vi "SPM Pump v0.1.vi"(0 "Delay before read (ms)":u32=1000, 1 "string to write":string="/1ZR", 2 "Time <input>":string, 3 "byte count":u32=64, 4 "Timeout (ms)":u32=10000, 5 "error in (no error)":errorcluster, 6 "Termination char\n(0xA = '\\n' = LF)\n(0xD = '\\r' = CR)":u8=13 format="%.0x", 7 "VISA resource name":refnum<visa-resource-name>="COM6", 10 "Enable Termination\nChar (T)":bool=TRUE, 11 "baud rate":u32=9600, 12 "parity":u16(ring) items=["None", "Odd", "Even", "Mark", "Space"], 13 "data bits":u16=8 min=5 max=8 step=1, 14 "stop bits":u16(ring)=10 items=["1.0"=10, "1.5"=15, "2.0"=20], 15 "flow control":u16(ring) items=["None"=0, "XON/XOFF"=1, "RTS/CTS"=2, "DTR/DSR"=4], 16 "Serial Settings:Serial End Mode for Reads":u16(ring)=2 items=["None", "LastBit", "TermChar"]) -> (8 "Error bit":string, 9 "Response":string, 18 "Serial port output":string, 19 "error out":errorcluster)   [LabVIEW 2016]
doc: "The Basic Serial Read and Write example performs a Serial Port Read, a Serial Port Write, or a combination of these actions. The user selects the actions (read or write) on the front panel. If both are selected, the VI will write the data first, read data, and then close the VISA session that is opened to the port. This VI will wait until the specified number of bytes is received at the port. Only the number of bytes specified will be read.\n\nINSTRUCTIONS:\n1) Select the serial resource and configuration parameters (baud rate, data bits, parity, stop bits, flow control).\n2) Select the operations to be performed. \n3) Connect the serial port to your device. If no device is available, perform a loopback test by doing one of the following. Short pins 2 and 3 on a RS-232 cable or short pin 4 to pin 8 and pin 5 to pin 9 on a RS-485/422 cable. \n4) Run the VI to see the data read. (The \"read string\" will match the \"string to write\" if a loopback test was performed.)\n\nNote: The parameters set for the serial port must match the parameters of the connected instrument or device. In this example, the bytes to read parameter specifies the number of bytes that the serial port reads. If there were more bytes at the port than the number specified in bytes to read, those bytes would not be read. Also, if you specify to read more bytes than the number of bytes actually read, you might receive a timeout error message.\n\nOn the block diagram, the Configure Serial Port VI sets the configuration parameters. The front panel displays the controls used to configure the basic parameters, such as baud rate, data bits, and parity. Constants configure the other parameters the user probably does not need set. After the VISA Configure Serial Port VI opens the VISA session and configures the port, the VI passes the VISA resource name to other VIs that perform operations on that VISA resource. The VISA Write function sends a command to the serial device and the VISA Read function returns data based on the command. The VISA Close function then closes the reference to the serial device. It is important to close the reference; otherwise communication through with that port through protocols other than VISA might not be possible."
panel:
  # "Select the serial resource and the operations (Read, Write, or both) to be performed.  If both are selected, the VI will write the data first, read data and then close the VISA session that is opened to the port.  This VI will wait until the specified number of bytes is received at the port. Only the number of bytes specified will be read."
  # "For additional information select File >> VI Properties >> Documentation"
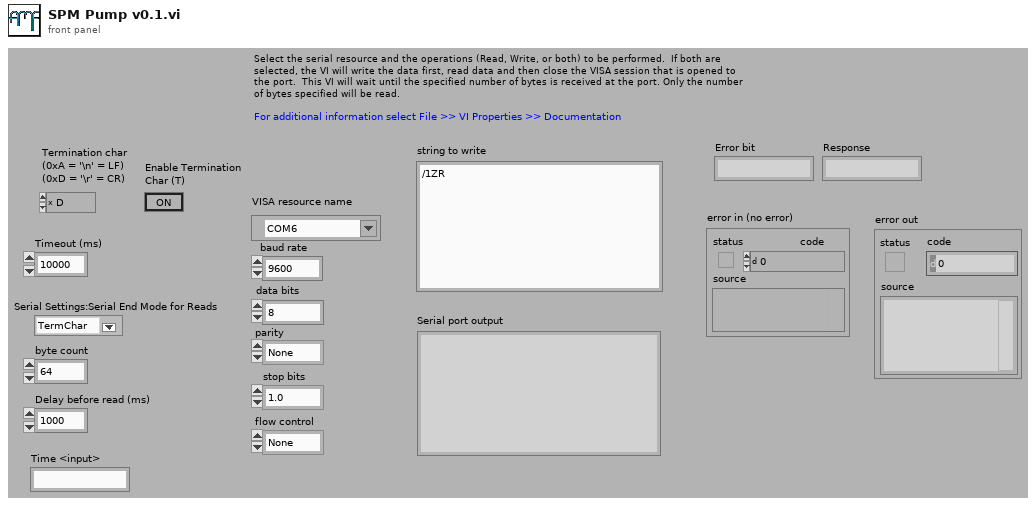
[diagram p1: front panel]
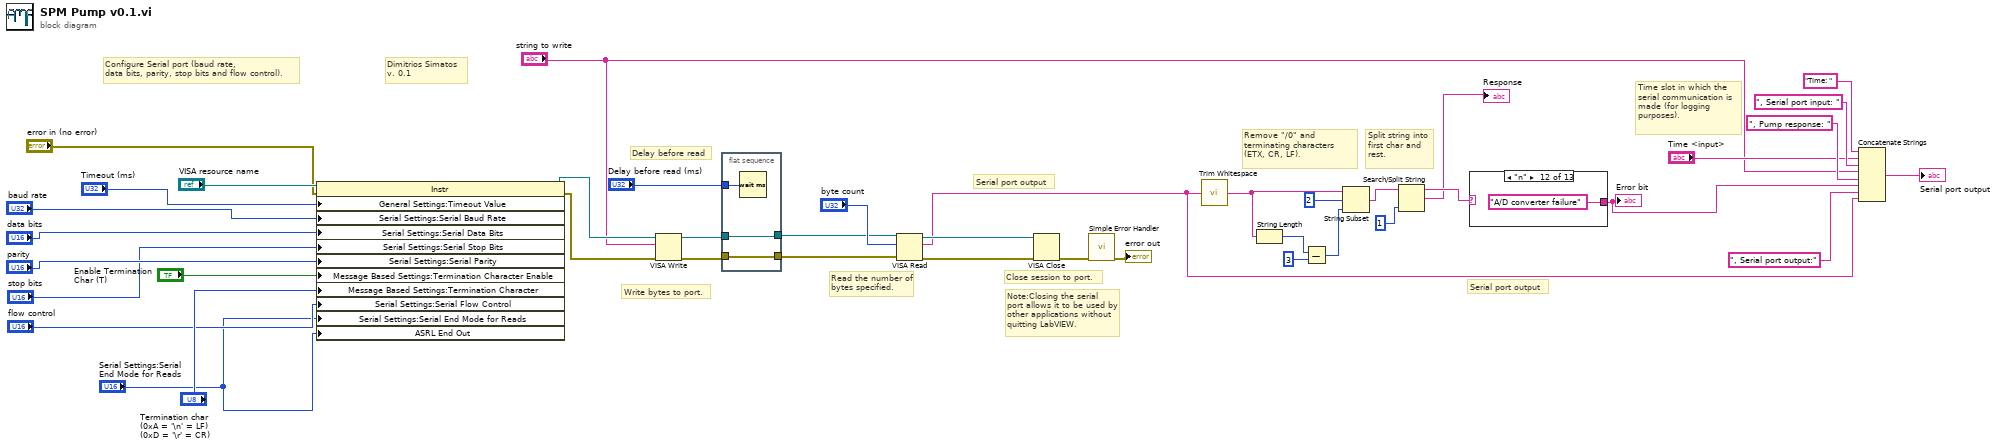
[diagram p0: block diagram]
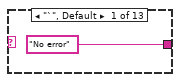
[diagram p2: hidden frame]
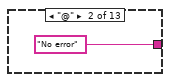
[diagram p3: hidden frame]
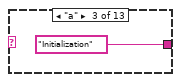
[diagram p4: hidden frame]
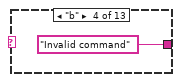
[diagram p5: hidden frame]
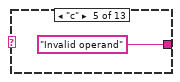
[diagram p6: hidden frame]
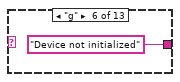
[diagram p7: hidden frame]
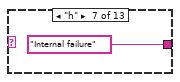
[diagram p8: hidden frame]
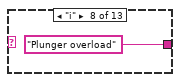
[diagram p9: hidden frame]
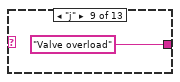
[diagram p10: hidden frame]
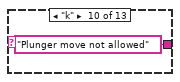
[diagram p11: hidden frame]
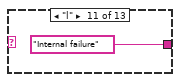
[diagram p12: hidden frame]
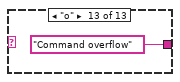
[diagram p13: hidden frame]
diagram:
  # "Serial port output"
  # "Serial port output"
  # "Time slot in which the serial communication is made (for logging purposes)."
  # "Split string into first char and rest."
  # "Remove \"/0\" and terminating characters (ETX, CR, LF)."
  # "Delay before read"
  # "Dimitrios Simatos\nv. 0.1"
  # "Read the number of bytes specified."
  # "Write bytes to port."
  # "Note:Closing the serial port allows it to be used by other applications without\nquitting LabVIEW."
  # "Configure Serial port (baud rate,\ndata bits, parity, stop bits and flow control)."
  # "Close session to port."
  n1 = property class="Instr"(reference="VISA resource name", error in="error in (no error)", "General Settings:Timeout Value"="Timeout (ms)", "Serial Settings:Serial Baud Rate"="baud rate", "Serial Settings:Serial Data Bits"="data bits", "Serial Settings:Serial Stop Bits"="stop bits", "Serial Settings:Serial Parity"="parity", "Message Based Settings:Termination Character Enable"="Enable Termination\nChar (T)", "Message Based Settings:Termination Character"="Termination char\n(0xA = '\\n' = LF)\n(0xD = '\\r' = CR)", "Serial Settings:Serial Flow Control"="flow control", "Serial Settings:Serial End Mode for Reads"="Serial Settings:Serial End Mode for Reads", "ASRL End Out"="Serial Settings:Serial End Mode for Reads") -> (reference out=w28:refnum<visa-resource-name>, error out=w27:errorcluster)
  n2 = VISA Write(VISA resource name=w28, write buffer="string to write", error in (no error)=w27) -> (VISA resource name out=w23:refnum<visa-resource-name>, error out=w22:errorcluster)  [unwired: 1 out]
  n3 = flat-sequence {
    tunnel: w22 -> [w43]
    tunnel: [w43] -> w21
    tunnel: w23 -> [w42]
    tunnel: [w42] -> w20
    tunnel: "Delay before read (ms)" -> [w44]
    frame #0 {
      n4 = Wait (ms)(milliseconds to wait=w44) -> ()  [unwired: 1 out]
    }
  }
  n5 = VISA Read(VISA resource name=w20, byte count="byte count", error in (no error)=w21) -> (VISA resource name out=w40:refnum<visa-resource-name>, read buffer=w3:string, error out=w41:errorcluster)  [unwired: 1 out]
  n6 = VISA Close(VISA resource name=w40, error in (no error)=w41) -> (error out=w39:errorcluster)
  n7 = call <vilib>:"Simple Error Handler.vi"("error in (no error)"=w39) -> ("error out"=→"error out":errorcluster)  [unwired: 4 in, 4 out]
  n8 = call <vilib>:"Trim Whitespace.vi"("string"=w3) -> ("trimmed string"=w14:string)  [unwired: 1 in]
  n9 = String Length(string=w14) -> (length=w18:i32)
  n10 = Subtract(x=w18, y=3) -> (x-y=w17:i32)
  n11 = String Subset(string=w14, offset (0)=2, length (rest)=w17) -> (substring=w13:string)
  n12 = Search/Split String(string=w13, offset (0)=1) -> (substring before match=w11:string, match + rest of string=→"Response":string)  [unwired: 1 in, 1 out]
  n13 = case shown="\"n\"" w11 {
    tunnel: ["No error" "No error" "Initialization" "Invalid command" "Invalid operand" "Device not initialized" "Internal failure" "Plunger overload" "Valve overload" "Plunger move not allowed" "Internal failure" "A/D converter failure" "Command overflow"] -> w4
    frame "`", Default {
    }
    frame "@" {
    }
    frame "a" {
    }
    frame "b" {
    }
    frame "c" {
    }
    frame "g" {
    }
    frame "h" {
    }
    frame "i" {
    }
    frame "j" {
    }
    frame "k" {
    }
    frame "l" {
    }
    frame "n" {
    }
    frame "o" {
    }
  }
  "Error bit" <- w4
  n14 = Concatenate Strings("Time: ", "Time <input>", ", Serial port input: ", "string to write", ", Pump response: ", w4, ", Serial port output:", w3) -> (→"Serial port output":string)
